vi "niDTS BT INSTR TX UTIL Channel Mode.vi"(7 "Chan Mode":enum16{"InBand", "Centered"}(ring)=enum."Centered") -> (8 "Chan Mode Parameter":enum16{"IBAnd", "CENTered"}(ring)=enum."CENTered")   [LabVIEW 2015, in "niDTS BT.lvlib" / "niDTS BT INSTR TX.lvclass"]
uses:
  niDTS BT INSTR TX.lvclass
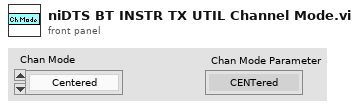
[diagram p1: front panel]
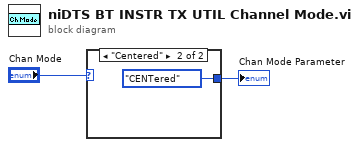
[diagram p0: block diagram]
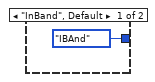
[diagram p2: hidden frame]
diagram:
  n1 = case shown="\"Centered\"" "Chan Mode" {
    tunnel: [enum16{"IBAnd", "CENTered"}."IBAnd" enum16{"IBAnd", "CENTered"}."CENTered"] -> w1
    frame "InBand", Default {
    }
    frame "Centered" {
    }
  }
  "Chan Mode Parameter" <- w1
